vi "AODO-Initialize DO Clock Source.vi"(0 "Sync Task":refnum<k21>, 5 "DAQmx Device Name":tag="PXI1Slot4", 7 "Fs (Hz)":dbl, 11 "error in (no error)":errorcluster) -> (4 "clock task":refnum<k21>, 15 "error out":errorcluster)   [LabVIEW 2020]
uses:
  <vilib>/DAQmx/create/channels.llb/DAQmx Create Channel (CO-Pulse Generation-Ticks).vi
  <vilib>/DAQmx/configure/timing.llb/DAQmx Timing (Implicit).vi
  <vilib>/DAQmx/configure/trigger.llb/DAQmx Start Trigger (Digital Edge).vi
  <resource>/objmgr/daqmx.rc
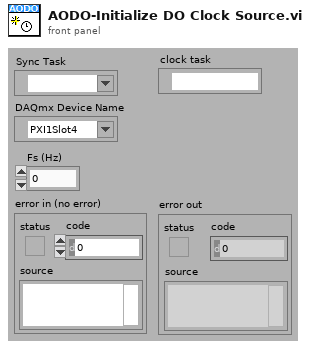
[diagram p1: front panel]
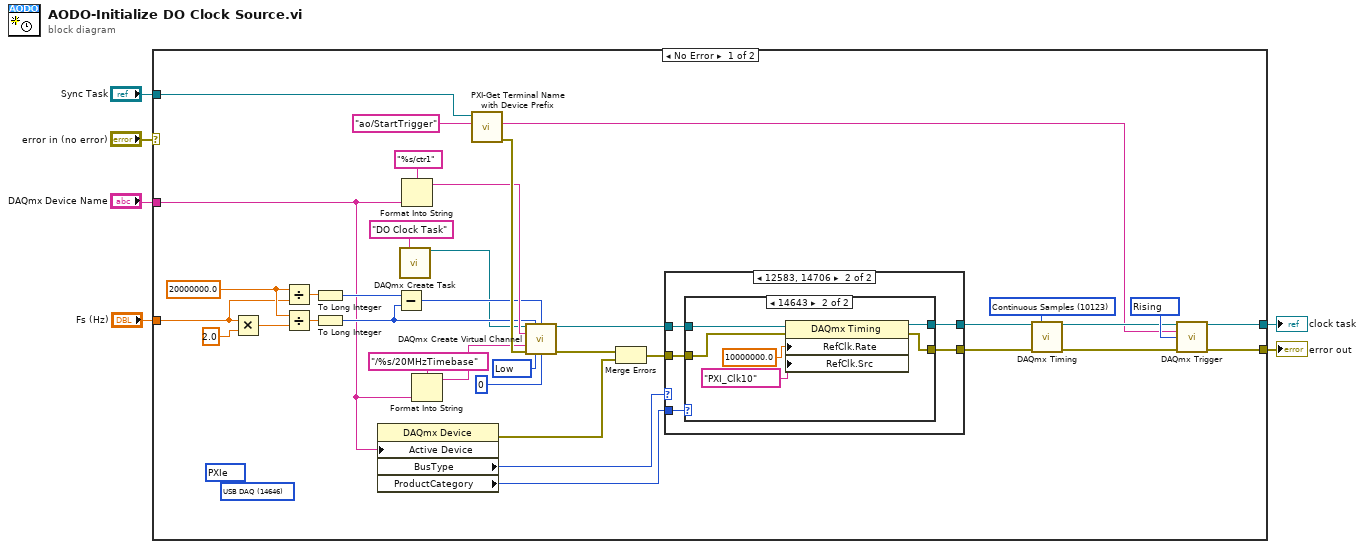
[diagram p0: block diagram]
diagram:
  n1 = case shown="No Error" "error in (no error)" {
    selector: "error in (no error)" -> [_ w58]
    tunnel: [w42 w58] -> w6
    tunnel: "DAQmx Device Name" -> [w17 _]
    tunnel: "Sync Task" -> [w16 _]
    tunnel: "Fs (Hz)" -> [w12 _]
    tunnel: [w15 _] -> w1
    frame No Error {
      (unwired) 14646 items=["M Series DAQ"=14643, "X Series DAQ"=15858, "E Series DAQ"=14642, "S Series DAQ"=14644, "B Series DAQ"=14662, "SC Series DAQ"=14645, "USB DAQ"=14646, "AO Series"=14647, "Digital I/O"=14648, "TIO Series"=14661, "Dynamic Signal Acquisition"=14649, "Switches"=14650, "CompactDAQ Chassis"=14658, "C Series Module"=14659, "SCXI Module"=14660, "SCC Connector Block"=14704, "SCC Module"=14705, "NI ELVIS"=14755, "Network DAQ"=14829, "SC Express"=15886, "Unknown"=12588] ("ProductCategory")
      (unwired) 14706 items=["PCI"=12582, "PCIe"=13612, "PXI"=12583, "PXIe"=14706, "SCXI"=12584, "SCC"=14707, "PCCard"=12585, "USB"=12586, "CompactDAQ"=14637, "TCP/IP"=14828, "Unknown"=12588, "SwitchBlock"=15870] ("BusType")
      w14 = 20000000.0 ("x")
      w26 = 10214 items=["High"=10192, "Low"=10214] ("idle state")
      w40 = 10280 items=["Rising"=10280, "Falling"=10171] ("Trigger Edge")
      w41 = 10123 items=["Finite Samples"=10178, "Continuous Samples"=10123] ("sample mode")
      n2 = Multiply(x=w12, y=2.0 ("x")) -> (x*y=w13:dbl)
      n3 = Divide(x=w14, y=w12) -> (x/y=w24:dbl)
      n4 = Divide(x=w14, y=w13) -> (x/y=w25:dbl)
      n5 = To Long Integer(number=w24) -> (32bit integer=w22:i32)
      n6 = To Long Integer(number=w25) -> (32bit integer=w23:i32)
      n7 = property class="DAQmx Device"("Active Device"=w17) -> (error out=w7:errorcluster, "BusType"=w19:i32, "ProductCategory"=w18:i32)  [unwired: 2 in, 1 out]
      n8 = Subtract(x=w22, y=w23) -> (x-y=w21:i32)
      n9 = call <vilib>:"DAQmx Create Task.vi"("new task name"="DO Clock Task" ("name to assign")) -> ("task out"=w9:refnum<k21>)  [unwired: 13 in, 1 out]
      n10 = Format Into String(format string="%s/ctr1", w17) -> (resulting string=w28:string)  [unwired: 2 in, 1 out]
      n11 = Format Into String(format string="/%s/20MHzTimebase", w17) -> (resulting string=w20:string)  [unwired: 2 in, 1 out]
      n12 = call "PXI-Get Terminal Name with Device Prefix.vi"("Local Terminal Name"="ao/StartTrigger", "task/channels in"=w16) -> ("error out"=w33:errorcluster, "Terminal Name with Device Prefix"=w34:string)  [unwired: 7 in, 1 out]
      n13 = call-poly <vilib>:"DAQmx Create Virtual Channel.vi"("task in"=w9, "high ticks"=w23, "low ticks"=w21, "counter"=w28, "source of ticks"=w20, "error in"=w33, "idle state"=w26, "initial delay"=u32 0) -> ("task out"=w31:refnum<k21>, "error out"=w32:errorcluster)  [unwired: 6 in]
      n14 = Merge Errors(w32, w7) -> (w8:errorcluster)
      n15 = case shown="12583, 14706" w19 {
        tunnel: [w44 w49] -> w38
        tunnel: [w43 w48] -> w37
        tunnel: w8 -> [w43 w47]
        tunnel: w31 -> [w44 w46]
        tunnel: w18 -> [_ w45]
        frame 0, Default {
        }
        frame 12583, 14706 {
          n16 = case shown="14643" w45 {
            tunnel: [w51 w57] -> w49
            tunnel: [w50 w56] -> w48
            tunnel: w47 -> [w50 w55]
            tunnel: w46 -> [w51 w54]
            frame 0, Default {
            }
            frame 14643 {
              n17 = property class="DAQmx Timing"(reference=w54, error in=w55, "RefClk.Rate"=10000000.0, "RefClk.Src"=tag "PXI_Clk10") -> (reference out=w57:refnum<k21>, error out=w56:errorcluster)
            }
          }
        }
      }
      n18 = call-poly <vilib>:"DAQmx Timing.vi"("task/channels in"=w38, "sample mode"=w41, "error in"=w37) -> ("task out"=w36:refnum<k21>, "error out"=w35:errorcluster)  [unwired: 11 in]
      n19 = call-poly <vilib>:"DAQmx Trigger.vi"("task/channels in"=w36, "source"=w34, "edge"=w40, "error in"=w35) -> ("task out"=w15:refnum<k21>, "error out"=w42:errorcluster)  [unwired: 10 in]
    }
    frame Error {
    }
  }
  "error out" <- w6
  "clock task" <- w1
